vi "SetCtlValue_Core.vi"(8 "error in (no error)":errorcluster, 9 "Value":variant, 10 "CtlName In":string, 11 "ctlRef_Maps in":refnum<class "ctlRef_Maps.lvclass">) -> (0 "error out":errorcluster, 3 "ctlRef_Maps out":refnum<class "ctlRef_Maps.lvclass">)   [LabVIEW 2020, in "CtlReferences.lvlib" / "ctlRef_Maps.lvclass"]
uses:
  ctlRef_Maps.lvclass
  C:/Viviota/Projects/R&D/VIV_ctlReferences/CtlReferences/CtlReferences.lvclass
  ctlRef_Maps.lvclass/ctlRef_Maps.ctl
  CtlReferences/CtlReferences.lvclass/CtlReferences.ctl
  CtlReferences/Read VIRef.vi
  CtlReferences/CtlReferences.lvclass
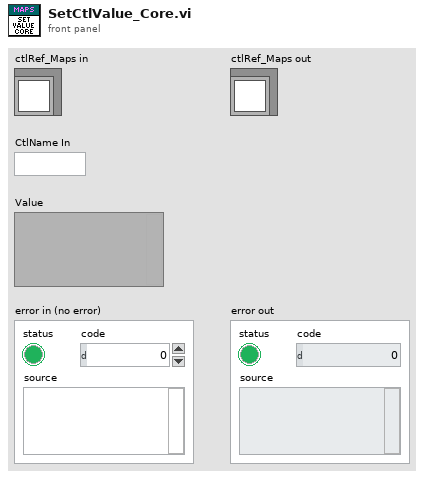
[diagram p1: front panel]
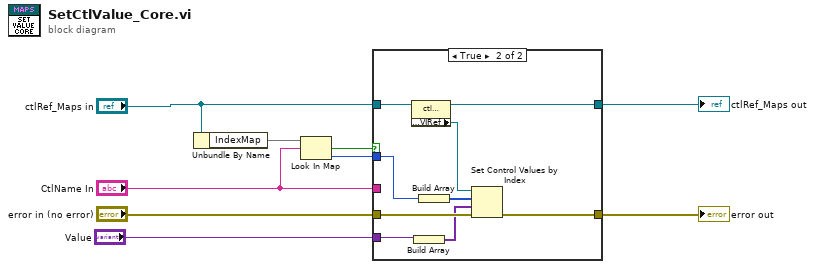
[diagram p0: block diagram]
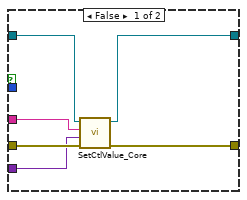
[diagram p2: hidden frame]
diagram:
  n1 = Unbundle By Name("ctlRef_Maps in") -> ("IndexMap"=w9:map{string, i32})
  n2 = Look In Map(map=w9, key="CtlName In") -> (key not found?=w8:bool, value=w7:i32)  [unwired: 1 in]
  n3 = case shown="True" w8 {
    tunnel: [w15 w16] -> w3
    tunnel: [w14 w20] -> w5
    tunnel: "error in (no error)" -> [w13 w23]
    tunnel: "ctlRef_Maps in" -> [w12 w24]
    tunnel: "CtlName In" -> [w11 _]
    tunnel: w7 -> [_ w22]
    tunnel: "Value" -> [w10 w18]
    frame False {
      n4 = call-parent "SetCtlValue_Core.vi"("error in (no error)"=w13, "Value"=w10, "CtlName In"=w11, "CtlReferences in"=w12) -> ("error out"=w15:errorcluster, "CtlReferences out"=w14:refnum<class "ctlRef_Maps.lvclass">)  [unwired: 6 in]
    }
    frame True {
      n5 = property class="ctlRef_Maps.lvclass"(reference=w24) -> (reference out=w20:refnum<class "ctlRef_Maps.lvclass">, "Accessors:VIRef"=w19:refnum<vi>)  [unwired: 1 in, 1 out]
      n6 = Build Array(w18) -> (w17:variant[])
      n7 = Build Array(w22) -> (w21:i32[])
      n8 = Set Control Values by Index(0:w19, 1:w21, 2:w17, 3:w23) -> (11:w16:errorcluster)
    }
  }
  "ctlRef_Maps out" <- w5
  "error out" <- w3
